vi "Integrate one peak (SubVI).vi"(0 "Time array":dbl[](array[numeric]), 1 "Start Index":i32, 2 "End Index":i32, 5 "Signal Array":dbl[](array[numeric]), 7 "Index cursor":dbl[](array[numeric]), 9 "Time cursor":dbl[](array[numeric]), 11 "Signal cursor":dbl[](array[numeric]), 15 "Lac standard area":dbl format="%.6e") -> (4 "Lac concentration":dbl format="%.4f", 12 "Lac area":dbl format="%.6e")   [LabVIEW 2014]
uses:
  <vilib>/Analysis/NI_AALPro.lvlib
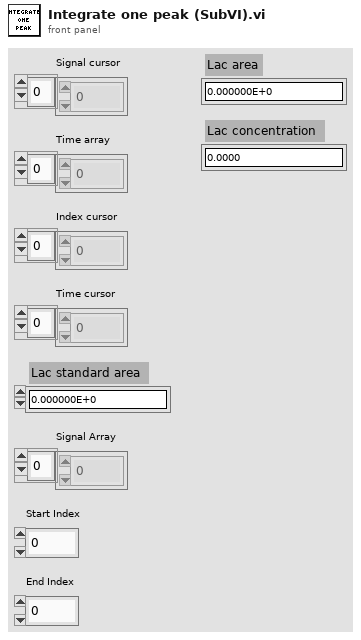
[diagram p1: front panel]
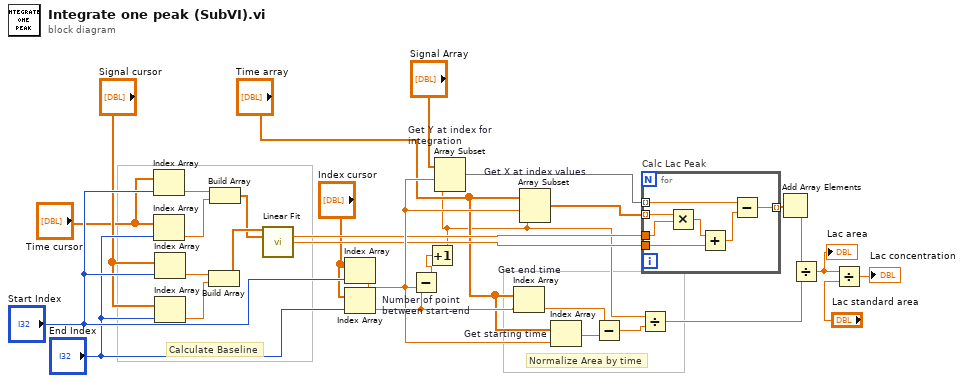
[diagram p0: block diagram]
diagram:
  # "Normalize Area by time"
  # "Calculate Baseline"
  n1 = Index Array(array="Time cursor", index="Start Index") -> (element=w6:dbl)
  n2 = Index Array(array="Time cursor", index="End Index") -> (element=w7:dbl)
  n3 = Index Array(array="Signal cursor", index="Start Index") -> (element=w8:dbl)
  n4 = Index Array(array="Signal cursor", index="End Index") -> (element=w9:dbl)
  n5 = Build Array(w8, w9) -> (w11:dbl[])
  n6 = Build Array(w6, w7) -> (w10:dbl[])
  n7 = call <vilib>:"Linear Fit.vi"("Y"=w11, "X"=w10) -> ("slope"=w20:dbl, "intercept"=w21:dbl)  [unwired: 9 in, 3 out]
  n8 = Index Array(array="Index cursor", index="Start Index") -> (element=w24:dbl)
  n9 = Index Array(array="Index cursor", index="End Index") -> (element=w25:dbl)
  n10 = Subtract "Number of point between start-end"(x=w25, y=w24) -> (x-y=w2:dbl)
  n11 = Increment(x=w2) -> (x+1=w1:dbl)
  n12 = Array Subset "Get Y at index for integration"(array="Signal Array", index=w24, length=w1) -> (w4:dbl[])
  n13 = Index Array "Get end time"(array="Time array", index=w25) -> (element=w18:dbl)
  n14 = Array Subset "Get X at index values"(array="Time array", index=w24, length=w1) -> (w15:dbl[])
  n15 = Index Array "Get starting time"(array="Time array", index=w24) -> (element=w17:dbl)
  n16 = Subtract(x=w18, y=w17) -> (x-y=w16:dbl)
  n17 = Divide(x=w1, y=w16) -> (x/y=w19:dbl)
  n18 = for "Calc Lac Peak" {
    tunnel: w15 -> [w37] mode=indexing
    tunnel: [w34] -> w23 mode=indexing
    tunnel: w20 -> [w33]
    tunnel: w21 -> [w32]
    tunnel: w4 -> [w31] mode=indexing
    n19 = Multiply(x=w37, y=w33) -> (x*y=w36:dbl)
    n20 = Add(x=w36, y=w32) -> (x+y=w35:dbl)
    n21 = Subtract(x=w31, y=w35) -> (x-y=w34:dbl)
  }
  n22 = Add Array Elements(numeric array=w23) -> (sum=w14:dbl)
  n23 = Divide(x=w14, y=w19) -> (x/y=w26:dbl)
  "Lac area" <- w26
  n24 = Divide(x=w26, y="Lac standard area") -> (x/y=→"Lac concentration":dbl)
